vi "Analysis.Selection.Get.vi"(7 "Action":enum8{"Get", "Set"}(ring), 8 "error in (no error)":errorcluster, 10 "Selections":T1={"Pull In Time"=TRUE, "Pull In Max Current"=TRUE, "Pull In Max Voltage"=TRUE, "Pull In Min Voltage"=TRUE, "Pull In Avg Voltage"=TRUE, "Hold Time"=TRUE, "Hold Max Current"=TRUE, "Hold Min Current"=TRUE, "Hold Avg Current"=TRUE, "Hold Max Voltage"=TRUE, "Hold Min Voltage"=TRUE, "Hold Avg Max Voltage"=TRUE, "Hold Avg Min Voltage"=TRUE, "Off Time"=TRUE, "Off Max Current"=TRUE, "Off Min Current"=TRUE, "Off Avg Current"=TRUE, "Off Max Voltage"=TRUE, "Off Min Voltage"=TRUE, "Off Avg Voltage"=TRUE, "Total Voltage Pulses"=TRUE, "Total Stage Time"=TRUE}, 11 "Item Ref in":T2 format="%.0x") -> (0 "error out":errorcluster, 2 "Selections":T1={"Pull In Time"=TRUE, "Pull In Max Current"=TRUE, "Pull In Max Voltage"=TRUE, "Pull In Min Voltage"=TRUE, "Pull In Avg Voltage"=TRUE, "Hold Time"=TRUE, "Hold Max Current"=TRUE, "Hold Min Current"=TRUE, "Hold Avg Current"=TRUE, "Hold Max Voltage"=TRUE, "Hold Min Voltage"=TRUE, "Hold Avg Max Voltage"=TRUE, "Hold Avg Min Voltage"=TRUE, "Off Time"=TRUE, "Off Max Current"=TRUE, "Off Min Current"=TRUE, "Off Avg Current"=TRUE, "Off Max Voltage"=TRUE, "Off Min Voltage"=TRUE, "Off Avg Voltage"=TRUE, "Total Voltage Pulses"=TRUE, "Total Stage Time"=TRUE}, 3 "Item Ref out":T2 format="%.0x")   [LabVIEW 2019, in "Fuel Injector Analysis Addon System Explorer.lvlib"]
uses:
  Fuel Injector Analysis Addon System Explorer.lvlib
  <vilib>/NI VeriStand/Custom Device API/Custom Device Item Ref.ctl
  Addon Shared/Types/Analysis.Channels.Select.ctl
  <vilib>/NI VeriStand/Custom Device API/Set Item Property (Boolean).vi
  <vilib>/NI VeriStand/Custom Device API/Get Item Property (Boolean).vi
  <vilib>/NI VeriStand/Custom Device API/Custom Device API.lvlib
  Addon Shared/Fuel Injector Analysis Addon Shared.lvlib
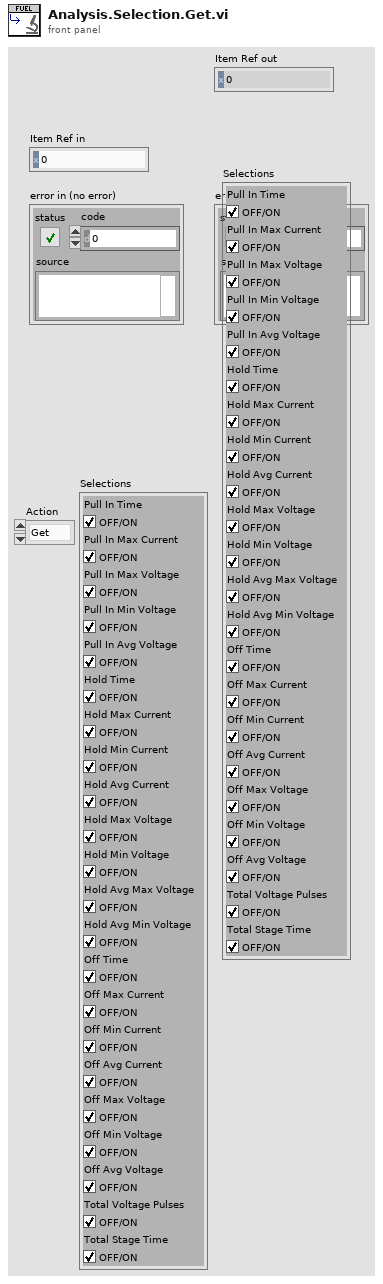
[diagram p1: front panel]
types:
  T1 = typedef "Fuel Injector Analysis Addon Shared.lvlib/Analysis.Channels.Select.ctl" = cluster{"Pull In Time":bool, "Pull In Max Current":bool, "Pull In Max Voltage":bool, "Pull In Min Voltage":bool, "Pull In Avg Voltage":bool, "Hold Time":bool, "Hold Max Current":bool, "Hold Min Current":bool, "Hold Avg Current":bool, "Hold Max Voltage":bool, "Hold Min Voltage":bool, "Hold Avg Max Voltage":bool, "Hold Avg Min Voltage":bool, "Off Time":bool, "Off Max Current":bool, "Off Min Current":bool, "Off Avg Current":bool, "Off Max Voltage":bool, "Off Min Voltage":bool, "Off Avg Voltage":bool, "Total Voltage Pulses":bool, "Total Stage Time":bool}
  T2 = typedef "Custom Device API.lvlib/Custom Device Item Ref.ctl" = u64
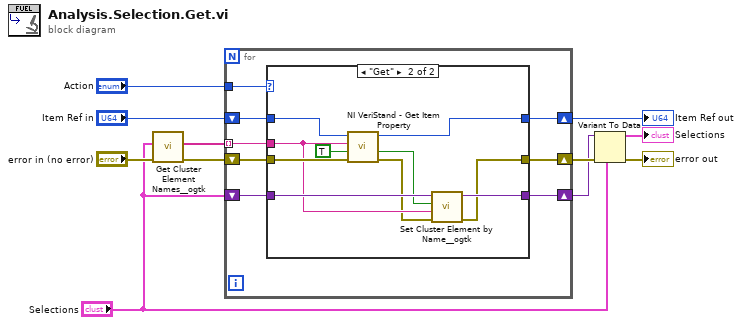
[diagram p0: block diagram]
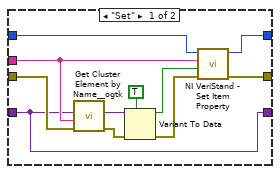
[diagram p2: hidden frame]
diagram:
  n1 = call <userlib>:"Get Cluster Element Names__ogtk.vi"("error in (no error)"="error in (no error)", "Cluster"="Selections") -> ("error out"=w8:errorcluster, "Element Names"=w7:string[])  [unwired: 8 in]
  n2 = for {
    shift-right: [w19] -> w11
    shift-left: "Item Ref in" -> [w18]
    shift-right: [w13] -> w6
    shift-left: w8 -> [w17]
    tunnel: w7 -> [w14] mode=indexing
    shift-right: [w15] -> w4
    shift-left: "Selections" -> [w16]
    tunnel: "Action" -> [w12]
    n3 = case shown="\"Get\"" w12 {
      tunnel: [w20 w40] -> w19
      tunnel: w18 -> [w30 w39]
      tunnel: w17 -> [w24 w38]
      tunnel: w16 -> [w21 w36]
      tunnel: [w21 w35] -> w15
      tunnel: w14 -> [w25 w34]
      tunnel: [w22 w31] -> w13
      frame "Set" {
        n4 = call <userlib>:"Get Cluster Element by Name__ogtk.vi"("error in (no error)"=w24, "Element Name"=w25, "Cluster"=w21) -> ("error out"=w28:errorcluster, "VElement"=w29:variant)  [unwired: 6 in, 1 out]
        n5 = Variant To Data(error in=w28, type=TRUE ("Default Value"), Variant=w29) -> (data=w26:bool, error out=w23:errorcluster)
        n6 = call-poly <vilib>:"NI VeriStand - Set Item Property.vi"("error in (no error)"=w23, "Value"=w26, "Property Name"=w25, "Item Ref in"=w30) -> ("error out"=w22:errorcluster, "Item Ref out"=w20:T2)  [unwired: 5 in, 1 out]
      }
      frame "Get" {
        n7 = call-poly <vilib>:"NI VeriStand - Get Item Property.vi"("error in (no error)"=w38, "Default Value"=TRUE, "Property Name"=w34, "Item Ref in"=w39) -> ("error out"=w32:errorcluster, "Value"=w33:bool, "Item Ref out"=w40:T2)  [unwired: 4 in, 1 out]
        n8 = call <userlib>:"Set Cluster Element by Name__ogtk.vi"("error in (no error)"=w32, "Element Name (\"\": New Element Data Name)"=w34, "New Element Value"=w33, "Cluster"=w36) -> ("error out"=w31:errorcluster, "VCluster out"=w35:variant)  [unwired: 5 in, 1 out]
      }
    }
  }
  "Item Ref out" <- w11
  n9 = Variant To Data(error in=w6, type="Selections", Variant=w4) -> (data=→"Selections":T1, error out=→"error out":errorcluster)
